vi "ex_FormatToCalcString.vi"(4 "number":dbl format="%#g") -> (1 "string":string)   [LabVIEW 2017]
doc: "Converts a number to its string representation."
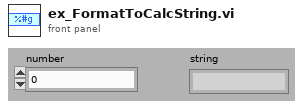
[diagram p1: front panel]
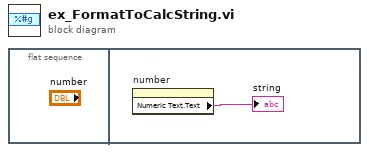
[diagram p0: block diagram]
diagram:
  n1 = flat-sequence {
    frame #0 {
    }
    frame #1 {
      n2 = property on="number" class="DigNum (strict)"() -> ("Numeric Text.Text"=→"string":string)  [unwired: 2 in, 2 out]
    }
  }
